vi "Test Time Zone Offset.vi"(8 "error in":errorcluster) -> (0 "error out":errorcluster)   [LabVIEW 2013]
uses:
  <vilib>/addons/_JKI Toolkits/Caraya/classes/Assert/Assert True.vi
  <vilib>/addons/_JKI Toolkits/Caraya/classes/Test/Test.lvclass
  <vilib>/addons/_JKI Toolkits/Caraya/classes/Assert/Assert.lvclass
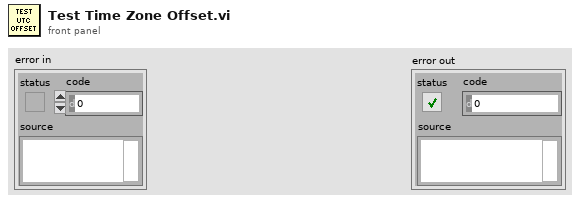
[diagram p1: front panel]
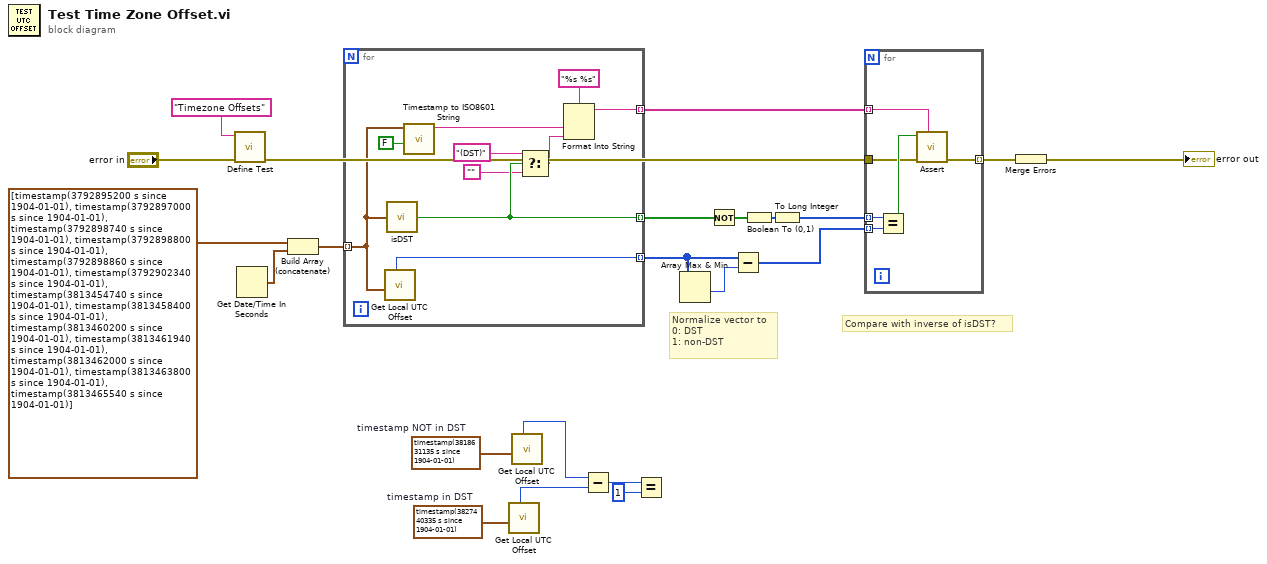
[diagram p0: block diagram]
diagram:
  w5 = timestamp(3818631135.0233965 s since 1904-01-01)  # timestamp NOT in DST
  w6 = timestamp(3827440335.0233965 s since 1904-01-01)  # timestamp in DST
  # "Compare with inverse of isDST?"
  # "Normalize vector to\n0: DST\n1: non-DST"
  n1 = call <vilib>:"Define Test.vi"("error in (no error)"="error in", "Label (VI Title)"="Timezone Offsets") -> ("error out"=w16:errorcluster)  [unwired: 8 in, 1 out]
  n2 = Get Date/Time In Seconds() -> (seconds since 1Jan1904=w20:timestamp)
  n3 = Build Array (concatenate)(timestamp[] [timestamp(3792895200 s since 1904-01-01), timestamp(3792897000 s since 1904-01-01), timestamp(3792898740 s since 1904-01-01), timestamp(3792898800 s since 1904-01-01), timestamp(3792898860 s since 1904-01-01), timestamp(3792902340 s since 1904-01-01), timestamp(3813454740 s since 1904-01-01), timestamp(3813458400 s since 1904-01-01), timestamp(3813460200 s since 1904-01-01), timestamp(3813461940 s since 1904-01-01), timestamp(3813462000 s since 1904-01-01), timestamp(3813463800 s since 1904-01-01), timestamp(3813465540 s since 1904-01-01)], w20) -> (w21:timestamp[])
  n4 = for {
    tunnel: w21 -> [w29] mode=indexing
    tunnel: [w27] -> w13 mode=indexing
    tunnel: [w28] -> w9 mode=indexing
    tunnel: [w23] -> w14 mode=indexing
    n5 = call "Get Local UTC Offset.vi"("timestamp (now)"=w29) -> ("UTC Offset (hours)"=w28:i32)  [unwired: 7 in, 3 out]
    n6 = call "isDST.vi"("timestamp (now)"=w29) -> ("is DST?"=w27:bool)  [unwired: 8 in]
    n7 = call "Timestamp to ISO8601 String.vi"("UTC? (F)"=FALSE, "Timestamp (now)"=w29) -> ("ISO8601 String"=w30:string)  [unwired: 9 in]
    n8 = Select(t="(DST)" ("format string"), s=w27, f="") -> (s? t:f=w25:string)
    n9 = Format Into String(format string="%s %s", w30, w25) -> (resulting string=w23:string)  [unwired: 2 in, 1 out]
  }
  n10 = call "Get Local UTC Offset.vi"("timestamp (now)"=w6) -> ("UTC Offset (hours)"=w4:i32)  [unwired: 7 in, 3 out]
  n11 = call "Get Local UTC Offset.vi"("timestamp (now)"=w5) -> ("UTC Offset (hours)"=w3:i32)  [unwired: 7 in, 3 out]
  n12 = Subtract(x=w3, y=w4) -> (x-y=w2:i32)
  n13 = Equal?(x=w2, y=1) -> ()  [unwired: 1 out]
  n14 = Array Max & Min(array=w9) -> (min value=w12:i32)  [unwired: 3 out]
  n15 = Not(x=w13) -> (.not. x?=w8:bool[])
  n16 = Subtract(x=w9, y=w12) -> (x-y=w10:i32[])
  n17 = Boolean To (0,1)(Boolean=w8) -> (0, 1=w11:i16[])
  n18 = To Long Integer(number=w11) -> (32bit integer=w7:i32[])
  n19 = for {
    tunnel: w7 -> [w38] mode=indexing
    tunnel: w10 -> [w37] mode=indexing
    tunnel: w16 -> [w35]
    tunnel: [w34] -> w15 mode=indexing
    tunnel: w14 -> [w33] mode=indexing
    n20 = Equal?(x=w38, y=w37) -> (x = y?=w36:bool)
    n21 = call-poly <vilib>:"Assert.vi"("Label"=w33, "error in (no error)"=w35, "True?"=w36) -> ("error out"=w34:errorcluster)  [unwired: 7 in, 1 out]
  }
  n22 = Merge Errors(w15) -> (→"error out":errorcluster)
